vi "Event Logger.vi"(8 "Error In":errorcluster, 11 "Event":T1 {"Time Stamp" format="%<%x %.3X>T"}) -> (0 "Error Out":errorcluster, 3 "Event out":T1 {"Time Stamp" format="%<%x %.3X>T"})   [LabVIEW 2019, in "GUI.lvlib"]
uses:
  GUI.lvlib
  Controls/Event.ctl
panel:
  in  "Filtered Error Codes":i32[](array[numeric])=[91, -314302]
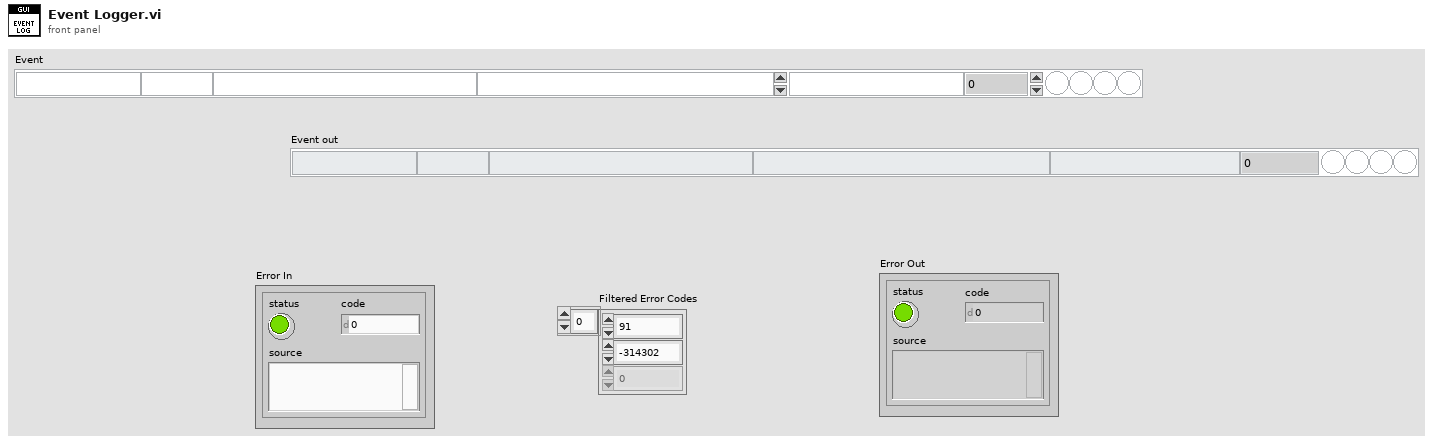
[diagram p1: front panel]
types:
  T1 = typedef "GUI.lvlib/Event.ctl" = cluster{"Name":string, "Time Stamp":timestamp, "Code":i32, "Source":string, "Value":string, "Boolean":bool, "Description":string, "Error":bool, "Warning":bool, " Fault":bool}
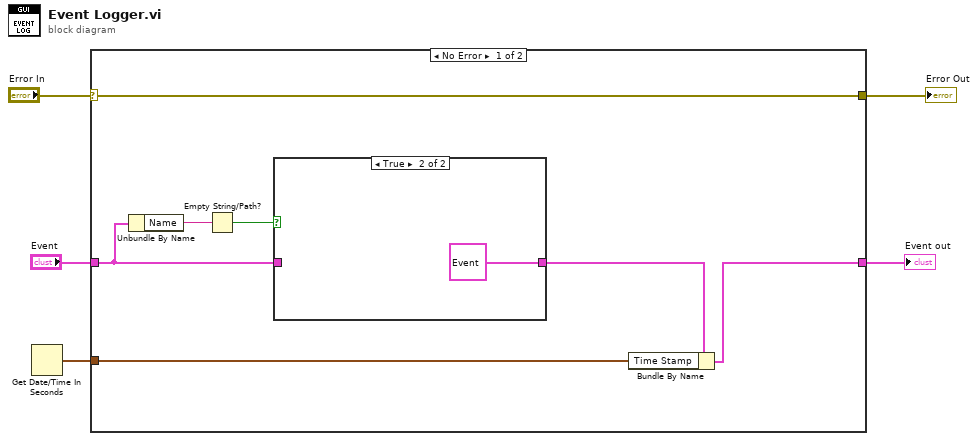
[diagram p0: block diagram]
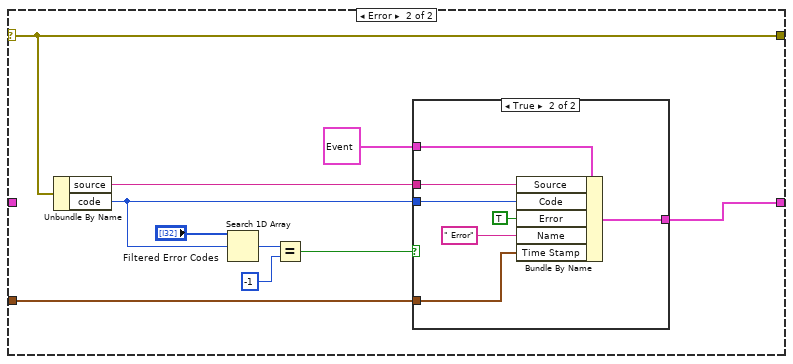
[diagram p3: hidden frame]
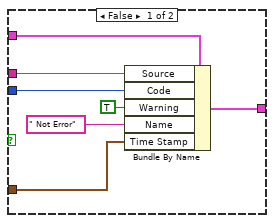
[diagram p4: hidden frame]
diagram:
  n1 = Get Date/Time In Seconds() -> (seconds since 1Jan1904=w1:timestamp)
  n2 = case shown="No Error" "Error In" {
    selector: "Error In" -> [w12 w19]
    tunnel: [w12 w19] -> w4
    tunnel: "Event" -> [w11 _]
    tunnel: [w7 w18] -> w2
    tunnel: w1 -> [w6 w16]
    frame No Error {
      n3 = Unbundle By Name(w11) -> ("Name"=w10:string)
      n4 = Empty String/Path?(string/path=w10) -> (empty?=w9:bool)
      n5 = case shown="True" w9 {
        tunnel: [w13 T1 {"Name"="", "Time Stamp"=timestamp(0 s since 1904-01-01), "Code"=0, "Source"="", "Value"="", "Boolean"=FALSE, "Description"="", "Error"=FALSE, "Warning"=FALSE, " Fault"=FALSE} ("Event")] -> w8
        tunnel: w11 -> [w13 _]
        frame False {
        }
        frame True {
        }
      }
      n6 = Bundle By Name(cluster=w8, "Time Stamp"=w6) -> (w7:T1)
    }
    frame Error {
      n7 = Unbundle By Name(w19) -> ("source"=w20:string, "code"=w17:i32)
      n8 = Search 1D Array(1D array="Filtered Error Codes", element=w17) -> (index of element=w23:i32)  [unwired: 1 out]
      n9 = Equal?(x=w23, y=-1) -> (x = y?=w21:bool)
      n10 = case shown="True" w21 {
        tunnel: w16 -> [w25 w32]
        tunnel: w20 -> [w29 w36]
        tunnel: [w28 w35] -> w18
        tunnel: w17 -> [w27 w34]
        tunnel: T1 {"Name"="", "Time Stamp"=timestamp(0 s since 1904-01-01), "Code"=0, "Source"="", "Value"="", "Boolean"=FALSE, "Description"="", "Error"=FALSE, "Warning"=FALSE, " Fault"=FALSE} ("Event") -> [w26 w33]
        frame False {
          n11 = Bundle By Name(cluster=w26, "Source"=w29, "Code"=w27, "Warning"=TRUE ("Error"), "Name"=" Not Error" ("string"), "Time Stamp"=w25) -> (w28:T1)
        }
        frame True {
          n12 = Bundle By Name(cluster=w33, "Source"=w36, "Code"=w34, "Error"=TRUE, "Name"=" Error" ("string"), "Time Stamp"=w32) -> (w35:T1)
        }
      }
    }
  }
  "Error Out" <- w4
  "Event out" <- w2
